vi "Read Position.vi"(8 "error in (no error)":errorcluster, 11 "Splitter in":refnum<class "Splitter.lvclass">) -> (0 "error out":errorcluster, 2 "Position":i32, 3 "Splitter out":refnum<class "Splitter.lvclass">)   [LabVIEW 2017, in "Splitter.lvclass"]
uses:
  Splitter.lvclass
  Splitter.lvclass/Splitter.ctl
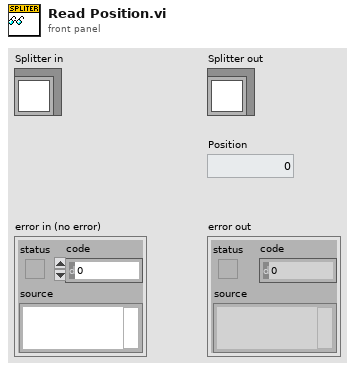
[diagram p1: front panel]
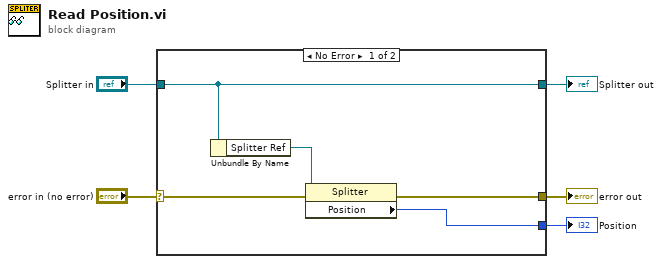
[diagram p0: block diagram]
diagram:
  n1 = case shown="No Error" "error in (no error)" {
    selector: "error in (no error)" -> [w10 w11]
    tunnel: [w8 w11] -> w4
    tunnel: [w9 w12] -> w2
    tunnel: "Splitter in" -> [w9 w12]
    tunnel: [w6 _] -> w1
    frame No Error {
      n2 = Unbundle By Name(w9) -> ("Splitter Ref"=w7:refnum<vi>)
      n3 = property class="Splitter"(reference=w7, error in=w10) -> (error out=w8:errorcluster, "Position"=w6:i32)  [unwired: 1 out]
    }
    frame Error {
    }
  }
  "error out" <- w4
  "Splitter out" <- w2
  "Position" <- w1
